vi "test-Diff-Drive-Accel-Limiter-Test2.vi"(8 "error in (no error)":errorcluster) -> (0 "error out":errorcluster, 3 "All tests passed":bool)   [LabVIEW 2019]
uses:
  <vilib>/Rock Robotics/WPI/ThirdParty/JAS_Junk/TrajLib/MatBuilder_Create.vi
  <vilib>/Rock Robotics/WPI/ThirdParty/JAS_Junk/TrajLib/LinearSystem_New.vi
  <vilib>/Rock Robotics/WPI/ThirdParty/JAS_Junk/TrajLib/MatrixHelper_Zero.vi
  <vilib>/Rock Robotics/WPI/ThirdParty/JAS_Junk/TrajLib/VecBuilder_2x1Fill.vi
  <vilib>/Analysis/baseanly.llb/A x B.vi
  <vilib>/Analysis/baseanly.llb/Real A x B.vi
  <vilib>/Rock Robotics/WPI/ThirdParty/JAS_Junk/TrajLib/Discretization_DiscretizeAB.vi
  <vilib>/Rock Robotics/WPI/ThirdParty/JAS_Junk/TrajLib/MatrixHelper_CoerceSize.vi
  <vilib>/Rock Robotics/WPI/ThirdParty/JAS_Junk/TrajLib/Matrix_Exp.vi
  <vilib>/Rock Robotics/WPI/ThirdParty/JAS_Junk/TrajLib/Matrix_AssignBlock.vi
  <vilib>/Rock Robotics/WPI/ThirdParty/JAS_Junk/TrajLib/Matrix_ExtractFrom.vi
  <vilib>/Analysis/7linalg.llb/Matrix Exp.vi
  <vilib>/Analysis/7linalg.llb/Real Matrix Exp.vi
  <vilib>/Analysis/Matrix/Numeric/Add/Add.vi
  <vilib>/Analysis/Matrix/Numeric/Add/Add - RM,RM.vi
  <vilib>/Analysis/7linalg.llb/Solve Linear Equations.vi
  <vilib>/Analysis/7linalg.llb/Solve Linear Equations (multiple right hand).vi
  <vilib>/Analysis/Matrix/Numeric/Subtract/Subtract.vi
  <vilib>/Analysis/Matrix/Numeric/Subtract/Subtract - RM,RM.vi
  <vilib>/Analysis/Matrix/Numeric/Multiply/Multiply.vi
  <vilib>/Analysis/Matrix/Numeric/Multiply/Multiply - RM,R.vi
  <vilib>/Rock Robotics/WPI/ThirdParty/JAS_Junk/TrajLib/Trajectory_Library.lvlib
panel:
  out "Test 1":bool
  out "Test 2":bool
  out "Test 3":bool
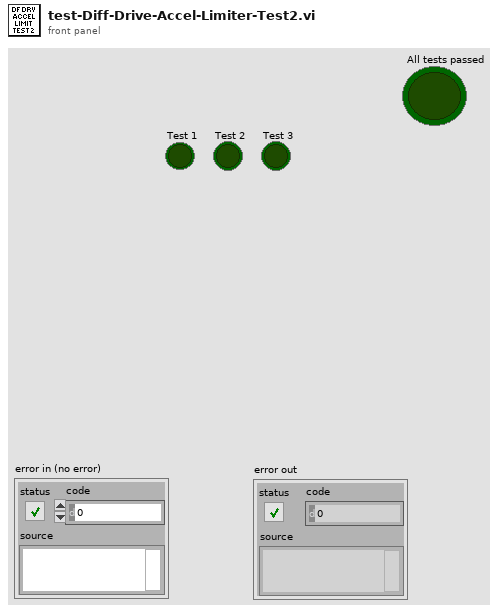
[diagram p1: front panel]
types:
  T1 = typedef "NI_Matrix.lvlib/RealMatrix.ctl" = dbl[][]
  T2 = typedef "Trajectory_Library.lvlib/LINEAR_SYSTEM.ctl" = cluster{"m_A":T1, "m_B":T1, "m_C":T1, "m_D":T1, "States":i32, "Inputs":i32, "Outputs":i32}
  T3 = typedef "Trajectory_Library.lvlib/DIFF_DRIVE_ACCEL_LIMIT.ctl" = cluster{"m_system":T2, "m_trackwidth":dbl, "m_maxLinearAccel":dbl, "m_maxAngularAccel":dbl, "m_minLinearAccel":dbl}
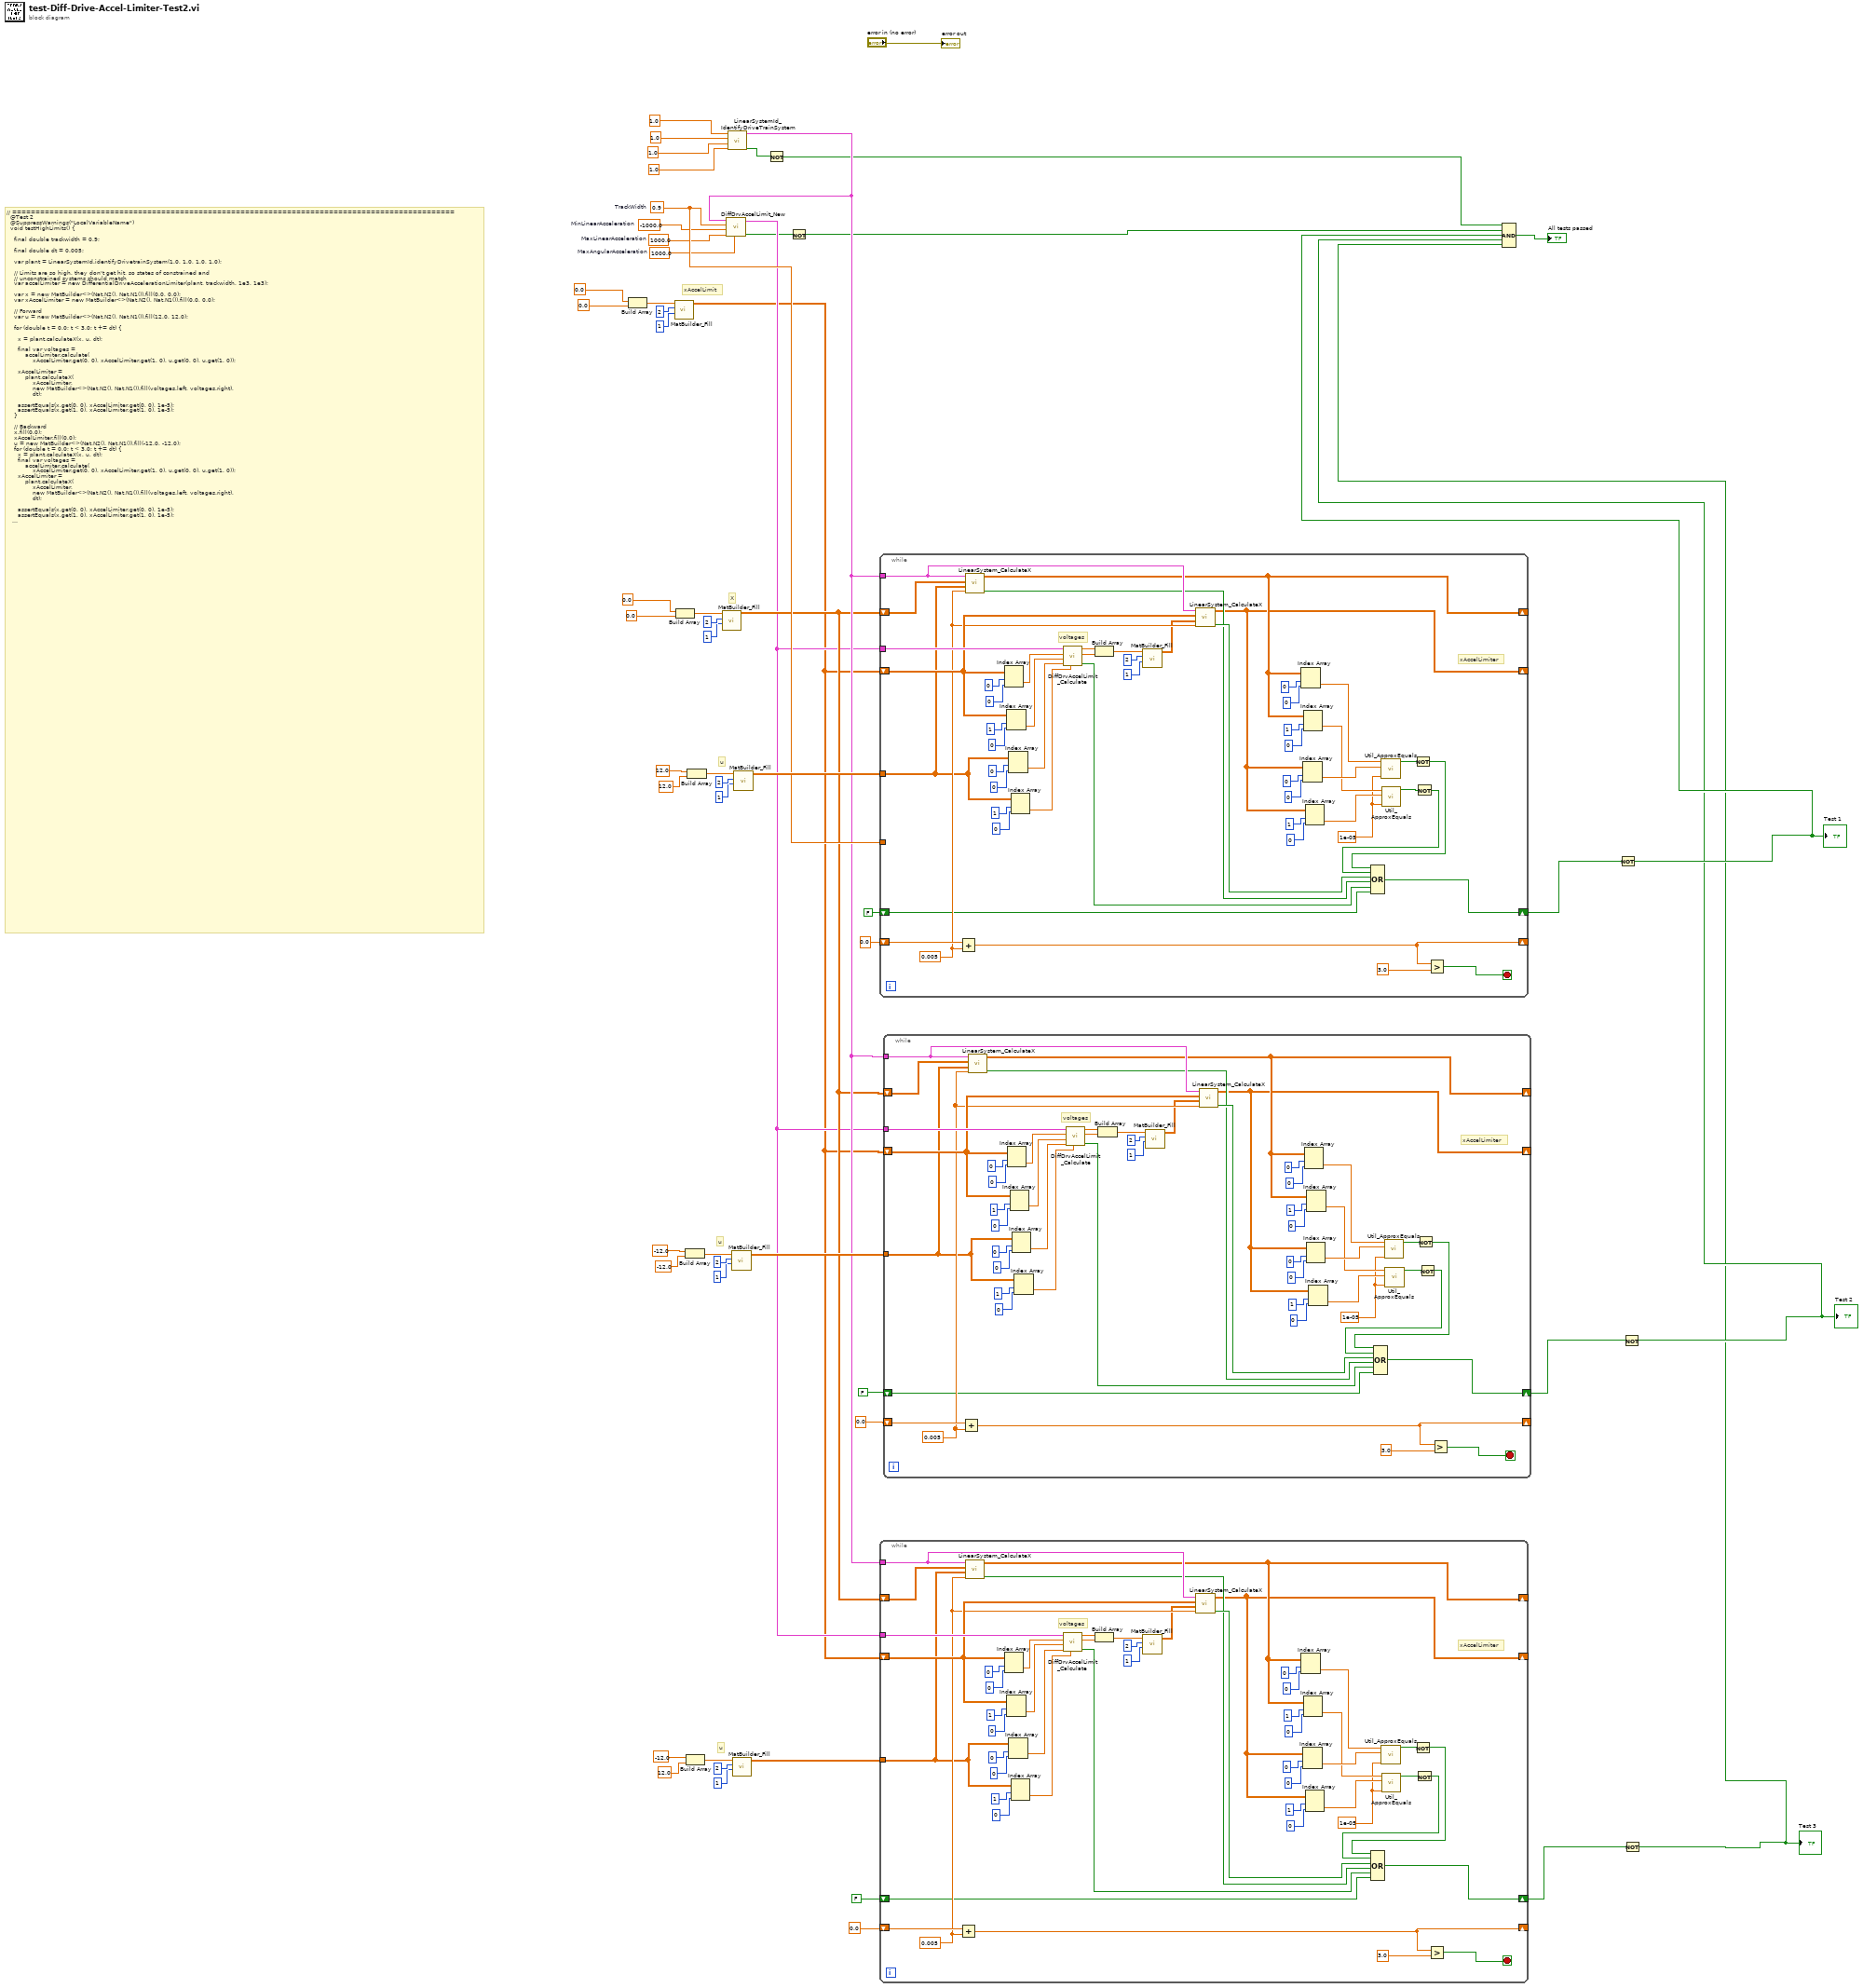
[diagram p0: block diagram]
diagram:
  w5 = -1000.0  # MinLinearAcceleration
  w24 = 0.9  # TrackWidth
  w6 = 1000.0  # MaxLinearAcceleration
  w7 = 1000.0  # MaxAngularAcceleration
  # "// ===============================================================================================\n  @Test 2\n  @SuppressWarnings(\"LocalVariableName\")\n  void testHighLimits() {\n\n    final double trackwidth = 0.9;\n\n    final double dt = 0.005;\n\n    var plant = LinearSystemId.identifyDrivetrainSystem(1.0, 1.0, 1.0, 1.0);\n\n    // Limits are so high, they don't get hit, so states of constrained and\n    // unconstrained systems should match\n    var accelLimiter = new DifferentialDriveAccelerationLimiter(plant, trackwidth, 1e3, 1e3);\n\n    var x = new MatBuilder<>(Nat.N2(), Nat.N1()).fill(0.0, 0.0);\n    var xAccelLimiter = new MatBuilder<>(Nat.N2(), Nat.N1()).fill(0.0, 0.0);\n\n    // Forward\n    var u = new MatBuilder<>(Nat.N2(), Nat.N1()).fill(12.0, 12.0);\n\n    for (double t = 0.0; t < 3.0; t += dt) {\n\n      x = plant.calculateX(x, u, dt);\n\n      final var voltages =\n          accelLimiter.calculate(\n              xAccelLimiter.get(0, 0), xAccelLimiter.get(1, 0), u.get(0, 0), u.get(1, 0));\n\n      xAccelLimiter =\n          plant.calculateX(\n              xAccelLimiter,\n              new MatBuilder<>(Nat.N2(), Nat.N1()).fill(voltages.left, voltages.right),\n              dt);\n\n      assertEquals(x.get(0, 0), xAccelLimiter.get(0, 0), 1e-5);\n      assertEquals(x.get(1, 0), xAccelLimiter.get(1, 0), 1e-5);\n    }\n\n    // Backward\n    x.fill(0.0);\n    xAccelLimiter.fill(0.0);\n    u = new MatBuilder<>(Nat.N2(), Nat.N1()).fill(-12.0, -12.0);\n    for (double t = 0.0; t < 3.0; t += dt) {\n      x = plant.calculateX(x, u, dt);\n      final var voltages =\n          accelLimiter.calculate(\n              xAccelLimiter.get(0, 0), xAccelLimiter.get(1, 0), u.get(0, 0), u.get(1, 0));\n      xAccelLimiter =\n          plant.calculateX(\n              xAccelLimiter,\n              new MatBuilder<>(Nat.N2(), Nat.N1()).fill(voltages.left, voltages.right),\n              dt);\n\n      assertEquals(x.get(0, 0), xAccelLimiter.get(0, 0), 1e-5);\n      assertEquals(x.get(1, 0), xAccelLimiter.get(1, 0), 1e-5);\n    }\n\n    // Rotate CCW\n    x.fill(0.0);\n    xAccelLimiter.fill(0.0);\n    u = new MatBuilder<>(Nat.N2(), Nat.N1()).fill(-12.0, 12.0);\n    for (double t = 0.0; t < 3.0; t += dt) {\n      x = plant.calculateX(x, u, dt);\n      final var voltages =\n          accelLimiter.calculate(\n              xAccelLimiter.get(0, 0), xAccelLimiter.get(1, 0), u.get(0, 0), u.get(1, 0));\n      xAccelLimiter =\n          plant.calculateX(\n              xAccelLimiter,\n              new MatBuilder<>(Nat.N2(), Nat.N1()).fill(voltages.left, voltages.right),\n              dt);\n\n      assertEquals(x.get(0, 0), xAccelLimiter.get(0, 0), 1e-5);\n      assertEquals(x.get(1, 0), xAccelLimiter.get(1, 0), 1e-5);\n    }\n  }\n}"
  # "u"
  # "u"
  # "u"
  # "xAccelLimit"
  # "X"
  n1 = Build Array(0.0 ("element"), 0.0 ("element")) -> (w48:dbl[])
  n2 = call <vilib>:"MatBuilder_Fill.vi"("Columns"=1, "Rows"=2, "Value List"=w48) -> ("output matrix"=w13:T1)  [unwired: 8 in]
  n3 = Build Array(0.0 ("element"), 0.0 ("element")) -> (w53:dbl[])
  n4 = Build Array(-12.0 ("element"), -12.0 ("element")) -> (w34:dbl[])
  n5 = Build Array(-12.0 ("element"), 12.0 ("element")) -> (w29:dbl[])
  n6 = Build Array(12.0 ("element"), 12.0 ("element")) -> (w43:dbl[])
  n7 = call <vilib>:"MatBuilder_Fill.vi"("Columns"=1, "Rows"=2, "Value List"=w53) -> ("output matrix"=w15:T1)  [unwired: 8 in]
  n8 = call <vilib>:"LinearSystemId_IdentifyDriveTrainSystem.vi"("kAAngular"=1.0 ("rbMeters"), "kVAngular"=1.0 ("rMeters"), "kALinear"=1.0 ("MassKg"), "kVLinear"=1.0 ("JKgMetersSquared")) -> ("Size Coerced"=w3:bool, "Linearsystem"=w16:T2)  [unwired: 6 in]
  n9 = call <vilib>:"DiffDrvAccelLimit_New.vi"("MaxAngularAcceleration"=w7, "MaxLinearAcceleration"=w6, "MinLinearAcceleration"=w5, "TrackWidth"=w24, "LINEARSYSTEM"=w16) -> ("Error"=w4:bool, "outDiffDriveAccelLimit"=w14:T3)  [unwired: 5 in]
  n10 = call <vilib>:"MatBuilder_Fill.vi"("Columns"=1, "Rows"=2, "Value List"=w34) -> ("output matrix"=w18:T1)  [unwired: 8 in]
  n11 = call <vilib>:"MatBuilder_Fill.vi"("Columns"=1, "Rows"=2, "Value List"=w29) -> ("output matrix"=w12:T1)  [unwired: 8 in]
  n12 = call <vilib>:"MatBuilder_Fill.vi"("Columns"=1, "Rows"=2, "Value List"=w43) -> ("output matrix"=w37:T1)  [unwired: 8 in]
  n13 = Not(x=w3) -> (.not. x?=w2:bool)
  n14 = Not(x=w4) -> (.not. x?=w1:bool)
  n15 = while {
    shift-right: [w107] -> _
    shift-left: 0.0 -> [w110]
    tunnel: w16 -> [w81]
    tunnel: w37 -> [w79]
    shift-right: [w69] -> _
    shift-left: w15 -> [w106]
    tunnel: w14 -> [w105]
    shift-right: [w68] -> _
    shift-left: w13 -> [w92]
    tunnel: w24 -> [_]
    shift-right: [w74] -> w35
    shift-left: FALSE -> [w75]
    stop <- w109 stop-if-true
    w63 = 1e-05 ("Tolerance")
    w86 = 0.005
    # "voltages"
    # "xAccelLimiter"
    n16 = Add(x=w110, y=w86) -> (x+y=w107:dbl)
    n17 = call <vilib>:"LinearSystem_CalculateX.vi"("dT_Seconds"=w86, "ClampedU"=w79, "X"=w106, "Linearsystem"=w81) -> ("Error"=w77:bool, "outX"=w69:T1)  [unwired: 6 in]
    n18 = Index Array(array=w92, index (row)=0, index (col)=0) -> (element=w100:dbl)
    n19 = Index Array(array=w92, index (row)=1, index (col)=0) -> (element=w99:dbl)
    n20 = Index Array(array=w79, index (row)=0, index (col)=0) -> (element=w94:dbl)
    n21 = Index Array(array=w79, index (row)=1, index (col)=0) -> (element=w93:dbl)
    n22 = call <vilib>:"DiffDrvAccelLimit_Calculate.vi"("RightVoltage"=w93, "LeftVoltage"=w94, "RightVelocity"=w99, "LeftVelocity"=w100, "inDiffDriveAccelLimit"=w105) -> ("Error"=w76:bool, "NewRightVoltage"=w87:dbl, "NewLeftVoltage"=w88:dbl)  [unwired: 4 in]
    n23 = Build Array(w88, w87) -> (w91:dbl[])
    n24 = call <vilib>:"MatBuilder_Fill.vi"("Columns"=1, "Rows"=2, "Value List"=w91) -> ("output matrix"=w80:T1)  [unwired: 8 in]
    n25 = call <vilib>:"LinearSystem_CalculateX.vi"("dT_Seconds"=w86, "ClampedU"=w80, "X"=w92, "Linearsystem"=w81) -> ("Error"=w78:bool, "outX"=w68:T1)  [unwired: 6 in]
    n26 = Index Array(array=w69, index (row)=0, index (col)=0) -> (element=w67:dbl)
    n27 = Index Array(array=w68, index (row)=0, index (col)=0) -> (element=w66:dbl)
    n28 = Index Array(array=w69, index (row)=1, index (col)=0) -> (element=w65:dbl)
    n29 = Index Array(array=w68, index (row)=1, index (col)=0) -> (element=w64:dbl)
    n30 = call <vilib>:"Util_ApproxEquals.vi"("Tolerance"=w63, "Value 2"=w66, "Value 1"=w67) -> ("ApproxEquals"=w61:bool)  [unwired: 8 in]
    n31 = call <vilib>:"Util_ApproxEquals.vi"("Tolerance"=w63, "Value 2"=w64, "Value 1"=w65) -> ("ApproxEquals"=w62:bool)  [unwired: 8 in]
    n32 = Not(x=w61) -> (.not. x?=w59:bool)
    n33 = Not(x=w62) -> (.not. x?=w60:bool)
    n34 = Compound Arithmetic op=OR(w59, w60, w78, w77, w76, w75) -> (w74:bool)
    n35 = Greater?(x=w107, y=3.0) -> (0:w109:bool)
  }
  n36 = while {
    shift-right: [w159] -> _
    shift-left: 0.0 -> [w162]
    tunnel: w16 -> [w133]
    tunnel: w12 -> [w131]
    shift-right: [w121] -> _
    shift-left: w15 -> [w158]
    tunnel: w14 -> [w157]
    shift-right: [w120] -> _
    shift-left: w13 -> [w144]
    shift-right: [w126] -> w9
    shift-left: FALSE -> [w127]
    stop <- w161 stop-if-true
    w115 = 1e-05 ("Tolerance")
    w138 = 0.005
    # "voltages"
    # "xAccelLimiter"
    n37 = Add(x=w162, y=w138) -> (x+y=w159:dbl)
    n38 = call <vilib>:"LinearSystem_CalculateX.vi"("dT_Seconds"=w138, "ClampedU"=w131, "X"=w158, "Linearsystem"=w133) -> ("Error"=w129:bool, "outX"=w121:T1)  [unwired: 6 in]
    n39 = Index Array(array=w144, index (row)=0, index (col)=0) -> (element=w152:dbl)
    n40 = Index Array(array=w144, index (row)=1, index (col)=0) -> (element=w151:dbl)
    n41 = Index Array(array=w131, index (row)=0, index (col)=0) -> (element=w146:dbl)
    n42 = Index Array(array=w131, index (row)=1, index (col)=0) -> (element=w145:dbl)
    n43 = call <vilib>:"DiffDrvAccelLimit_Calculate.vi"("RightVoltage"=w145, "LeftVoltage"=w146, "RightVelocity"=w151, "LeftVelocity"=w152, "inDiffDriveAccelLimit"=w157) -> ("Error"=w128:bool, "NewRightVoltage"=w139:dbl, "NewLeftVoltage"=w140:dbl)  [unwired: 4 in]
    n44 = Build Array(w140, w139) -> (w143:dbl[])
    n45 = call <vilib>:"MatBuilder_Fill.vi"("Columns"=1, "Rows"=2, "Value List"=w143) -> ("output matrix"=w132:T1)  [unwired: 8 in]
    n46 = call <vilib>:"LinearSystem_CalculateX.vi"("dT_Seconds"=w138, "ClampedU"=w132, "X"=w144, "Linearsystem"=w133) -> ("Error"=w130:bool, "outX"=w120:T1)  [unwired: 6 in]
    n47 = Index Array(array=w121, index (row)=0, index (col)=0) -> (element=w119:dbl)
    n48 = Index Array(array=w120, index (row)=0, index (col)=0) -> (element=w118:dbl)
    n49 = Index Array(array=w121, index (row)=1, index (col)=0) -> (element=w117:dbl)
    n50 = Index Array(array=w120, index (row)=1, index (col)=0) -> (element=w116:dbl)
    n51 = call <vilib>:"Util_ApproxEquals.vi"("Tolerance"=w115, "Value 2"=w118, "Value 1"=w119) -> ("ApproxEquals"=w113:bool)  [unwired: 8 in]
    n52 = call <vilib>:"Util_ApproxEquals.vi"("Tolerance"=w115, "Value 2"=w116, "Value 1"=w117) -> ("ApproxEquals"=w114:bool)  [unwired: 8 in]
    n53 = Not(x=w113) -> (.not. x?=w111:bool)
    n54 = Not(x=w114) -> (.not. x?=w112:bool)
    n55 = Compound Arithmetic op=OR(w111, w112, w130, w129, w128, w127) -> (w126:bool)
    n56 = Greater?(x=w159, y=3.0) -> (0:w161:bool)
  }
  n57 = while {
    shift-right: [w211] -> _
    shift-left: 0.0 -> [w214]
    tunnel: w16 -> [w185]
    tunnel: w18 -> [w183]
    shift-right: [w173] -> _
    shift-left: w15 -> [w210]
    tunnel: w14 -> [w209]
    shift-right: [w172] -> _
    shift-left: w13 -> [w196]
    shift-right: [w178] -> w21
    shift-left: FALSE -> [w179]
    stop <- w213 stop-if-true
    w167 = 1e-05 ("Tolerance")
    w190 = 0.005
    # "voltages"
    # "xAccelLimiter"
    n58 = Add(x=w214, y=w190) -> (x+y=w211:dbl)
    n59 = call <vilib>:"LinearSystem_CalculateX.vi"("dT_Seconds"=w190, "ClampedU"=w183, "X"=w210, "Linearsystem"=w185) -> ("Error"=w181:bool, "outX"=w173:T1)  [unwired: 6 in]
    n60 = Index Array(array=w196, index (row)=0, index (col)=0) -> (element=w204:dbl)
    n61 = Index Array(array=w196, index (row)=1, index (col)=0) -> (element=w203:dbl)
    n62 = Index Array(array=w183, index (row)=0, index (col)=0) -> (element=w198:dbl)
    n63 = Index Array(array=w183, index (row)=1, index (col)=0) -> (element=w197:dbl)
    n64 = call <vilib>:"DiffDrvAccelLimit_Calculate.vi"("RightVoltage"=w197, "LeftVoltage"=w198, "RightVelocity"=w203, "LeftVelocity"=w204, "inDiffDriveAccelLimit"=w209) -> ("Error"=w180:bool, "NewRightVoltage"=w191:dbl, "NewLeftVoltage"=w192:dbl)  [unwired: 4 in]
    n65 = Build Array(w192, w191) -> (w195:dbl[])
    n66 = call <vilib>:"MatBuilder_Fill.vi"("Columns"=1, "Rows"=2, "Value List"=w195) -> ("output matrix"=w184:T1)  [unwired: 8 in]
    n67 = call <vilib>:"LinearSystem_CalculateX.vi"("dT_Seconds"=w190, "ClampedU"=w184, "X"=w196, "Linearsystem"=w185) -> ("Error"=w182:bool, "outX"=w172:T1)  [unwired: 6 in]
    n68 = Index Array(array=w173, index (row)=0, index (col)=0) -> (element=w171:dbl)
    n69 = Index Array(array=w172, index (row)=0, index (col)=0) -> (element=w170:dbl)
    n70 = Index Array(array=w173, index (row)=1, index (col)=0) -> (element=w169:dbl)
    n71 = Index Array(array=w172, index (row)=1, index (col)=0) -> (element=w168:dbl)
    n72 = call <vilib>:"Util_ApproxEquals.vi"("Tolerance"=w167, "Value 2"=w170, "Value 1"=w171) -> ("ApproxEquals"=w165:bool)  [unwired: 8 in]
    n73 = call <vilib>:"Util_ApproxEquals.vi"("Tolerance"=w167, "Value 2"=w168, "Value 1"=w169) -> ("ApproxEquals"=w166:bool)  [unwired: 8 in]
    n74 = Not(x=w165) -> (.not. x?=w163:bool)
    n75 = Not(x=w166) -> (.not. x?=w164:bool)
    n76 = Compound Arithmetic op=OR(w163, w164, w182, w181, w180, w179) -> (w178:bool)
    n77 = Greater?(x=w211, y=3.0) -> (0:w213:bool)
  }
  n78 = Not(x=w35) -> (.not. x?=w22:bool)
  "Test 1" <- w22
  n79 = Not(x=w21) -> (.not. x?=w17:bool)
  "Test 2" <- w17
  n80 = Not(x=w9) -> (.not. x?=w8:bool)
  "Test 3" <- w8
  n81 = Compound Arithmetic op=AND(w2, w1, w22, w17, w8) -> (→"All tests passed":bool)
  "error out" <- "error in (no error)"
